vi "AA-Lockin_Save.vi"(8 "error in (no error)":errorcluster, 9 "Finished?":bool, 11 "SweepControl.lvclass":refnum<class "SweepControl.lvclass">) -> (0 "error out":errorcluster)   [LabVIEW 2016, in "Transport.lvclass"]
uses:
  Transport.lvclass
  <userlib>/LevyLab/Lockin-Multichannel/Typedefs/AO-cluster.ctl
  <userlib>/LevyLab/Lockin-Multichannel/Typedefs/AO_Amp-array.ctl
  <userlib>/LevyLab/Lockin-Multichannel/Typedefs/AO_DC-array.ctl
  <userlib>/LevyLab/Lockin-Multichannel/Typedefs/AO_f-array.ctl
  <userlib>/LevyLab/Lockin-Multichannel/Typedefs/AO_phi-array.ctl
  <userlib>/LevyLab/Lockin-Multichannel/Typedefs/Function-array.ctl
  <userlib>/LevyLab/Lockin-Multichannel/Typedefs/Function-enum.ctl
  SMOs/SweepControl/SweepControl.lvclass
  <userlib>/LevyLab/Levylab Instruments/Instrument.lvclass
  <userlib>/LevyLab/LV to ITX/LVtoITX.lvclass
  Control Experiment/Control Experiment.lvclass
panel:
  in  "Tab Control":enum32{"lockin/SG Control", "Data"}(tab)
  in  "Channels: AO":T1={"AO amp (V)"=[0.0002, 0.0, 0.0, 0.0, 0.0, 0.0, 0.0, 0.0], "AO DC (V)"=[0.00025, 0.0, 0.0, 0.0, 0.0, 0.0, 0.0, 0.0], "AO f (Hz)"=[13.0, 13.0, 13.0, 13.0, 13.0, 13.0, 13.0, 13.0], "AO phi (°)"=[0.0, 0.0, 0.0, 0.0, 0.0, 0.0, 0.0, 0.0], "function"=[enum."Sine", enum."Sine", enum."Sine", enum."Sine", enum."Sine", enum."Sine", enum."Sine", enum."Sine"], "I+"=[]} {"AO f (Hz)" min=0.001 max=10000.0; "AO DC (V)" format="%.3p"; "AO amp (V)" format="%.3p"}
  out "Vmax (end)":dbl=0.7 format="%#_3p"
  out "Vmin (start)":dbl=-0.15 format="%#_3p"
  out "dV":dbl=0.0005 format="%#_3p"
  in  "Comments":string="SA03036H\nsweep Vsg:-150m to 700m, 500u steps\nB 7T to -7T\nVbg =-3.9V\nT: 50mK\n\nlockin\n\nI+/-: 4/28 200uV ac+ 250u dc bias, 13Hz\nV1+/-: 3/27\nV2+/- 2/6\nV3+/V3-: 7/8\nVsg: 1\nVbg :26\n\ntc 300ms order 2"
  in  "ITX folder":string="4L4Lockinfieldsweep"
  out "T (mK)":dbl
  in  "wait after setting Vsg (ms)":u32
  in  "Initial wait (ms)":u32=10000
  out "side gate channel":i32=1
  in  "Physical Channel":tag="Dev2/ao0" caption="Back Gate Channel"
  in  "Sweep":enum16{"Vsg", "Vbg"}(ring)
  in  "cycles (1,2,...)":i32=1 min=1 step=1
  in  "phase":dbl
  out "ramp rate":dbl=0.2 format="%#_13g"
  out "Field":dbl=0.5 format="%#_13g"
  in  "function (ramp)":enum16{"Ramp", "Triangle", "Sine"}(ring)
  in  "set \"Vsg\" to initial value?":bool
  out "time (ms)":u32=76
  out "G 4T":cluster{"Y":dbl[], "Y":dbl[]}[](graph)
  out "Lockins":cluster{"Y":dbl[], "Y":dbl[]}[](graph)
  out "Lockins 2":cluster{"Y":dbl[], "Y":dbl[]}[](graph)
  # "1"
  # "2"
  # "3"
  # "4"
  # "5"
  # "6"
  # "7"
  # "8"
  # "dynamically name the traces"
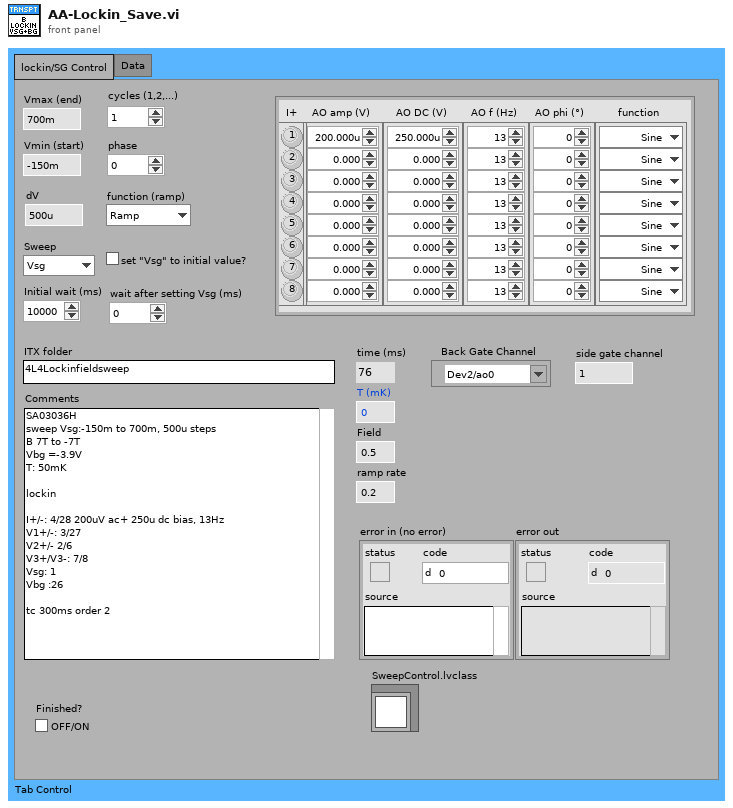
[diagram p1: front panel]
types:
  T1 = typedef "AO-cluster.ctl" = cluster{"AO amp (V)":T2, "AO DC (V)":T3, "AO f (Hz)":T4, "AO phi (°)":T5, "function":T6, "I+":bool[]}
  T2 = typedef "AO_Amp-array.ctl" = dbl[]
  T3 = typedef "AO_DC-array.ctl" = dbl[]
  T4 = typedef "AO_f-array.ctl" = dbl[]
  T5 = typedef "AO_phi-array.ctl" = dbl[]
  T6 = typedef "Function-array.ctl" = T7[]
  T7 = typedef "Function-enum.ctl" = enum16{"Sine", "Triangle", "Square", "Sawtooth"}
  T8 = typedef "SweepControl.lvclass/ScanParamters.ctl" = T9[]
  T9 = typedef "SweepControl.lvclass/Cluster - ScanParamters.ctl" = cluster{"Start":dbl, "End":dbl, "Step":dbl, "Rate":dbl, "wait (ms)":u32, "address":refnum<visa-resource-name>, "Channel":i32}
  T10 = typedef "Control Experiment.lvclass/Control Experiment FGV-cluster.ctl" = cluster{"path":path, "device":string, "user":string, "comments":string, "Lockin Ch":enum16{"1", "2", "3", "4", "5", "6", "7", "8"}[], "Electrode":u32[], "Label":string[], "KH Ch":enum32{"1", "2", "3", "4", "5", "6", "7", "8"}[], "Configuration":enum16{"Ground", "Current", "Voltage", "Gate"}[], "Gain":u32[], "Shunt Resistor":u32[]}
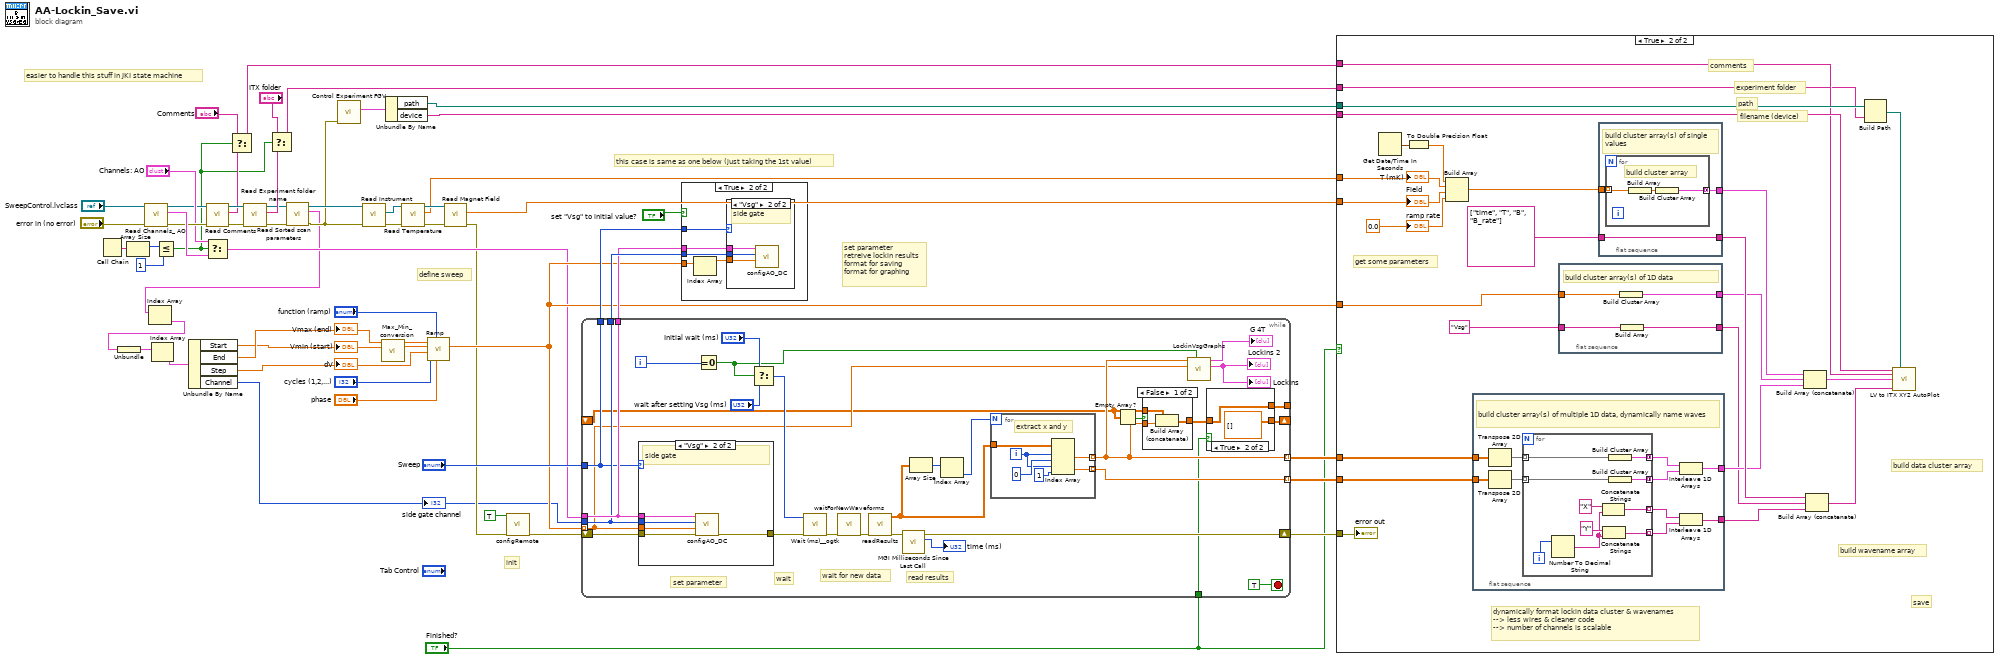
[diagram p0: block diagram]
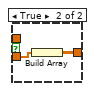
[diagram p3: hidden frame]
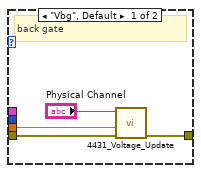
[diagram p5: hidden frame]
diagram:
  # "easier to handle this stuff in JKI state machine"
  # "define sweep"
  # "set parameter\nretreive lockin results\nformat for saving\nformat for graphing"
  # "this case is same as one below (just taking the 1st value)"
  # "init"
  n1 = Call Chain() -> (call chain=w42:string[])
  n2 = Array Size(array=w42) -> (size(s)=w41:i32)
  n3 = call-dynamic "Read Channels_ AO.vi"("error in (no error)"="error in (no error)", "SweepControl in"="SweepControl.lvclass") -> ("error out"=w34:errorcluster, "Channels: AO"=w39:T1, "SweepControl out"=w32:refnum<class "SweepControl.lvclass">)  [unwired: 7 in]
  n4 = Less Or Equal?(x=w41, y=1) -> (x <= y?=w22:bool)
  n5 = call-dynamic "Read Comments.vi"("error in (no error)"=w34, "SweepControl in"=w32) -> ("error out"=w36:errorcluster, "Comments"=w24:string, "SweepControl out"=w35:refnum<class "SweepControl.lvclass">)  [unwired: 7 in]
  n6 = Select(t="Channels: AO", s=w22, f=w39) -> (s? t:f=w37:T1)
  n7 = Select(t="Comments", s=w22, f=w24) -> (s? t:f=w19:string)
  n8 = call-dynamic "Read Experiment folder name.vi"("error in (no error)"=w36, "SweepControl in"=w35) -> ("error out"=w5:errorcluster, "Experiment folder name"=w23:string, "SweepControl out"=w4:refnum<class "SweepControl.lvclass">)  [unwired: 7 in]
  n9 = Select(t="ITX folder", s=w22, f=w23) -> (s? t:f=w18:string)
  n10 = call-dynamic "Read Sorted scan parameters.vi"("error in (no error)"=w5, "SweepControl in"=w4) -> ("error out"=w2:errorcluster, "Sorted scan parameters"=w1:cluster{T8}[], "SweepControl out"=w3:refnum<class "SweepControl.lvclass">)  [unwired: 7 in]
  n11 = Index Array(array=w1) -> (element=w15:cluster{T8})  [unwired: 1 in]
  n12 = Unbundle(w15) -> (w16:T8)
  n13 = Index Array(array=w16) -> (element=w14:T9)  [unwired: 1 in]
  n14 = Unbundle By Name(w14) -> ("Start"=w11:dbl, "End"=w13:dbl, "Step"=w12:dbl, "Channel"=w10:i32)
  "dV" <- w12
  "Vmax (end)" <- w13
  "Vmin (start)" <- w11
  "side gate channel" <- w10
  n15 = call "Control Experiment FGV.vi"("error in (no error)"=w2) -> ("Cluster out"=w8:T10)  [unwired: 9 in, 1 out]
  n16 = call-dynamic "Read Instrument.vi"("error in (no error)"=w2, "SweepControl in"=w3) -> ("error out"=w26:errorcluster, "Instrument.lvclass"=w25:refnum<class "Instrument.lvclass">)  [unwired: 7 in, 1 out]
  n17 = call <userlib>:"Max_Min_conversion.vi"("Min"=w11, "Max"=w13) -> ("offset"=w56:dbl, "Amplitude"=w57:dbl)  [unwired: 8 in]
  n18 = Unbundle By Name(w8) -> ("path"=w6:path, "device"=w7:string)
  n19 = call-dynamic "Read Temperature.vi"("error in (no error)"=w26, "Instrument in"=w25) -> ("error out"=w27:errorcluster, "Temperature (K)"=w30:dbl, "Instrument out"=w31:refnum<class "Instrument.lvclass">)  [unwired: 6 in, 1 out]
  n20 = call <userlib>:"Ramp.vi"("phase"="phase", "function (ramp)"="function (ramp)", "cycles (1,2,...)"="cycles (1,2,...)", "step size"=w12, "offset"=w56, "amplitude"=w57) -> ("Waveform Graph"=w44:dbl[])  [unwired: 3 in, 2 out]
  n21 = call-dynamic "Read Magnet Field.vi"("error in (no error)"=w27, "Instrument in"=w31) -> ("error out"=w17:errorcluster, "Field (T)"=w29:dbl)  [unwired: 6 in, 2 out]
  n22 = call <userlib>:"configRemote.vi"("error in (no error)"=w17, "Remote Mode"=TRUE) -> ("error out"=w50:errorcluster)  [unwired: 9 in]
  n23 = while {
    tunnel: w37 -> [w88]
    tunnel: w44 -> [w61] mode=indexing
    tunnel: "Sweep" -> [w86]
    tunnel: w10 -> [w87]
    tunnel: [w88] -> w49
    tunnel: [w87] -> w52
    tunnel: [w86] -> w51
    shift-right: [w82] -> w45
    shift-left: w50 -> [w85]
    tunnel: [w66] -> w47 mode=indexing
    tunnel: [w67] -> w46 mode=indexing
    shift-right: [w63] -> _
    shift-left: _ -> [w59]
    tunnel: "Finished?" -> [w65]
    tunnel: [w62] -> _
    i -> [w83]
    stop <- TRUE stop-if-true
    # "read results"
    # "wait for new data"
    # "wait"
    # "set parameter"
    n24 = case shown="\"Vsg\"" w86 {
      tunnel: w88 -> [_ w111]
      tunnel: w61 -> [w106 w109]
      tunnel: w87 -> [_ w110]
      tunnel: w85 -> [w104 w108]
      tunnel: [w103 w107] -> w84
      frame "Vbg", Default {
        # "back gate"
        n25 = call "4431_Voltage_Update.vi"("error in"=w104, "Amplified output"=w106, "Physical Channel(s)"="Physical Channel") -> ("error out"=w103:errorcluster)  [unwired: 8 in]
      }
      frame "Vsg" {
        # "side gate"
        n26 = call <userlib>:"configAO_DC.vi"("error in (no error)"=w108, "new DC (V)"=w109, "AO Channel"=w110, "Channels: AO"=w111) -> ("error out"=w107:errorcluster)  [unwired: 6 in, 1 out]
      }
    }
    n27 = Equal To 0?(x=w83) -> (x = 0?=w71:bool)
    n28 = Select(t="Initial wait (ms)", s=w71, f="wait after setting Vsg (ms)") -> (s? t:f=w74:u32)
    n29 = call <userlib>:"Wait (ms)__ogtk.vi"("error in (no error)"=w84, "milliseconds to wait"=w74) -> ("error out"=w77:errorcluster)  [unwired: 8 in, 1 out]
    n30 = call <userlib>:"waitForNewWaveforms.vi"("error in (no error)"=w77) -> ("error out"=w72:errorcluster)  [unwired: 9 in, 1 out]
    n31 = call <userlib>:"readResults.vi"("error in (no error)"=w72) -> ("error out"=w81:errorcluster, "Results"=w80:dbl[][])  [unwired: 8 in, 1 out]
    n32 = call <userlib>:"MGI Milliseconds Since Last Call.vi"("Error In"=w81) -> ("ms"=→"time (ms)":u32, "Error Out"=w82:errorcluster)  [unwired: 5 in]
    n33 = Array Size(array=w80) -> (size(s)=w79:i32[])
    n34 = Index Array(array=w79) -> (element=w78:i32)  [unwired: 1 in]
    n35 = for {
      N: w78 -> [_]
      tunnel: w80 -> [w100]
      tunnel: [w98] -> w66 mode=indexing
      tunnel: [w97] -> w67 mode=indexing
      i -> [w99]
      # "extract x and y"
      n36 = Index Array(array=w100, index (row) #1=w99, index (col) #1=0 ("disabled index (col)"), index (row) #2=w99, index (col) #2=1 ("disabled index (col)")) -> (element #1=w98:dbl, element #2=w97:dbl)
    }
    n37 = Empty Array?(array=w59) -> (empty?=w60:bool)
    n38 = case shown="False" w60 {
      tunnel: w66 -> [w91 w93]
      tunnel: [w90 w92] -> w64
      tunnel: w59 -> [w89 _]
      frame False {
        n39 = Build Array (concatenate)(w89, w91) -> (w90:dbl[][])
      }
      frame True {
        n40 = Build Array(w93) -> (w92:dbl[][])
      }
    }
    n41 = call "LockinVsgGraphs.vi"("reset?"=w71, "paramter in"=w61, "Y array in"=w66) -> ("Y vs X"=→"Lockins" →"Lockins 2":cluster{"Y":dbl[], "Y":dbl[]}[], "Array out"=→"G 4T":cluster{"Y":dbl[], "Y":dbl[]}[])  [unwired: 7 in]
    n42 = case shown="True" w65 {
      tunnel: w64 -> [w94 w95]
      tunnel: [w94 dbl[][] []] -> w63
      tunnel: [w94 w95] -> w62
      frame False {
      }
      frame True {
      }
    }
  }
  n43 = case shown="True" "set \"Vsg\" to initial value?" {
    tunnel: w49 -> [_ w116]
    tunnel: w44 -> [_ w115]
    tunnel: w52 -> [_ w113]
    tunnel: w51 -> [_ w114]
    frame False {
    }
    frame True {
      n44 = Index Array(array=w115) -> (element=w112:dbl)  [unwired: 1 in]
      n45 = case shown="\"Vsg\"" w114 {
        tunnel: w116 -> [_ w117]
        tunnel: w112 -> [_ w118]
        tunnel: w113 -> [_ w119]
        frame "Vbg", Default {
          # "back gate"
        }
        frame "Vsg" {
          # "side gate"
          n46 = call <userlib>:"configAO_DC.vi"("new DC (V)"=w118, "AO Channel"=w119, "Channels: AO"=w117) -> ()  [unwired: 7 in, 2 out]
        }
      }
    }
  }
  n47 = case shown="True" "Finished?" {
    tunnel: w47 -> [_ w143]
    tunnel: w46 -> [_ w142]
    tunnel: w45 -> [_ w120]
    tunnel: w44 -> [_ w127]
    tunnel: w30 -> [_ w126]
    tunnel: w29 -> [_ w125]
    tunnel: w7 -> [_ w124]
    tunnel: w6 -> [_ w123]
    tunnel: w19 -> [_ w122]
    tunnel: w18 -> [_ w121]
    frame False {
    }
    frame True {
      w130 = 0.0
      # "filename (device)"
      # "path"
      # "comments"
      # "experiment folder"
      # "get some parameters"
      # "save"
      # "build data cluster array"
      # "build wavename array"
      # "dynamically format lockin data cluster & wavenames\n--> less wires & cleaner code\n--> number of channels is scalable"
      n48 = Get Date/Time In Seconds() -> (seconds since 1Jan1904=w133:timestamp)
      n49 = To Double Precision Float(number=w133) -> (double precision float=w131:dbl)
      n50 = Build Array(w131, w126, w125, w130) -> (w132:dbl[])
      n51 = flat-sequence {
        tunnel: w143 -> [w158]
        tunnel: w142 -> [w157]
        tunnel: [w150] -> w137
        tunnel: [w149] -> w136
        frame #0 {
          # "build cluster array(s) of multiple 1D data, dynamically name waves"
          n52 = Transpose 2D Array(2D array=w158) -> (transposed array=w156:dbl[][])
          n53 = Transpose 2D Array(2D array=w157) -> (transposed array=w155:dbl[][])
          n54 = for {
            tunnel: w156 -> [w168] mode=indexing
            tunnel: w155 -> [w167] mode=indexing
            tunnel: [w166] -> w154 mode=concatenating
            tunnel: [w165] -> w153 mode=concatenating
            tunnel: [w160] -> w152 mode=indexing
            tunnel: [w159] -> w151 mode=indexing
            i -> [w162]
            n55 = Number To Decimal String(number=w162) -> (decimal integer string=w161:string)  [unwired: 1 in]
            n56 = Concatenate Strings("X" ("wavenames"), w161) -> (w160:string)
            n57 = Concatenate Strings("Y" ("wavenames"), w161) -> (w159:string)
            n58 = Build Cluster Array(w168) -> (w166:cluster{dbl[]}[])
            n59 = Build Cluster Array(w167) -> (w165:cluster{dbl[]}[])
          }
          n60 = Interleave 1D Arrays(w154, w153) -> (w149:cluster{dbl[]}[])
          n61 = Interleave 1D Arrays(w152, w151) -> (w150:string[])
        }
      }
      n62 = flat-sequence {
        tunnel: [w145] -> w135
        tunnel: w127 -> [w148]
        tunnel: [w147] -> w134
        tunnel: "Vsg" ("wavenames") -> [w146]
        frame #0 {
          # "build cluster array(s) of 1D data"
          n63 = Build Cluster Array(w148) -> (w147:cluster{"Waveform Graph":dbl[]}[])
          n64 = Build Array(w146) -> (w145:string[])
        }
      }
      n65 = flat-sequence {
        tunnel: [w171] -> w140
        tunnel: [w169] -> w138
        tunnel: w132 -> [w170]
        tunnel: string[] ["time", "T", "B", "B_rate"] ("wavenames (.Vx, etc)") -> [w169]
        frame #0 {
          # "build cluster array(s) of single values"
          n66 = for {
            tunnel: [w173] -> w171 mode=concatenating
            tunnel: w170 -> [w172] mode=indexing
            # "build cluster array"
            n67 = Build Array(w172) -> (w174:dbl[])
            n68 = Build Cluster Array(w174) -> (w173:cluster{dbl[]}[])
          }
        }
      }
      n69 = Build Array (concatenate)(w140, w134, w136) -> (w139:cluster{"Waveform Graph":dbl[]}[])
      n70 = Build Array (concatenate)(w138, w135, w137) -> (w141:string[])
      n71 = Build Path(base path=w123, name or relative path=w121) -> (appended path=w144:path)
      n72 = call <userlib>:"LV to ITX XY2 AutoPlot.vi"("filename"=w124, "path"=w144, "Notes"=w122, "Data"=w139, "wavenames (.Vx, etc)"=w141) -> ()  [unwired: 10 in, 1 out]
      "T (mK)" <- w126
      "ramp rate" <- w130
      "Field" <- w125
      "error out" <- w120
    }
  }
